vi "Find Request In VI.vi"(7 "Memory in (empty":path[](array[path]), 8 "error in":errorcluster, 10 "Level (0)":i32, 11 "VI Ref":refnum<vi>) -> (0 "error out":errorcluster, 2 "Request And Wait For Reply Names":string[](array[string]), 3 "Request Names":string[](array[string]), 5 "Memory out":path[](array[path]))   [LabVIEW 2021, in "TAF Proj Document Type.lvlib" / "Project Parser.lvlib"]
uses:
  <vilib>/Wovalab/AntiDoc/Document Type/Add-ons/LabVIEW TAF Project/Project Parser/Project Parser.lvlib
  <vilib>/Utility/traverseref.llb/TRef TravTarget.ctl
  <vilib>/Utility/traverseref.llb/VI Scripting - Traverse.lvlib
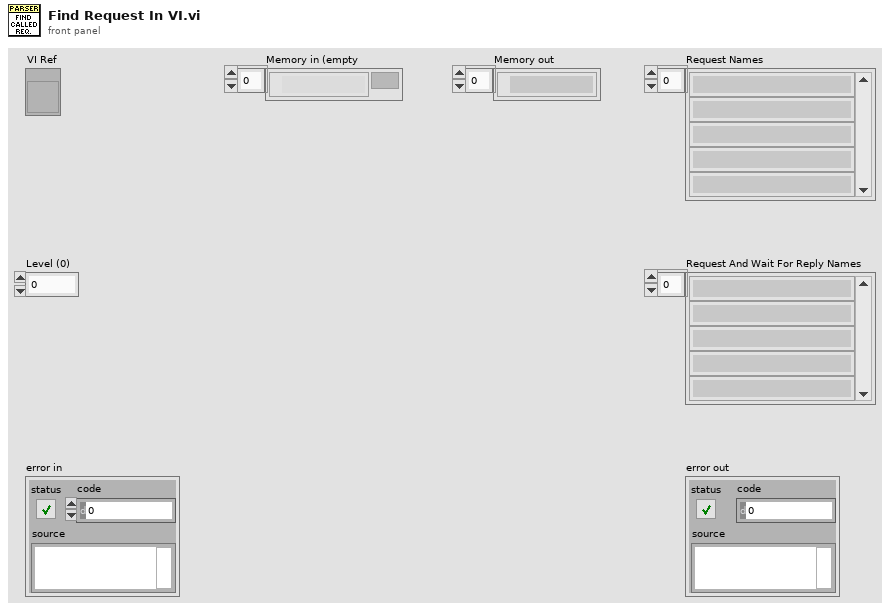
[diagram p1: front panel]
types:
  T1 = typedef "TRef TravTarget.ctl" = enum16{"FP", "BD", "Other"}
  T2 = typedef "TAF Proj Document Type.lvlib/Project Parser.lvlib/Dqmh Event Type--enum.ctl" = enum16{"Not a DQMH Event", "Request", "Request And Wait For Reply", "Broadcast"}
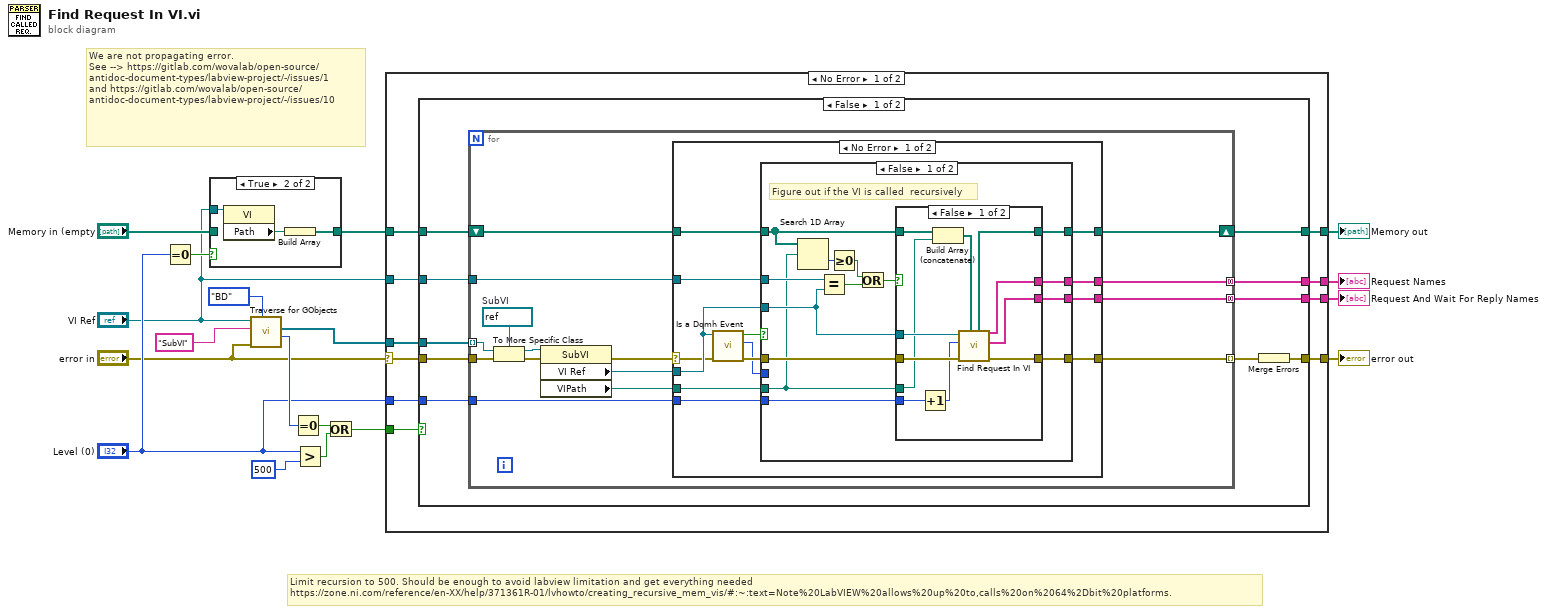
[diagram p0: block diagram]
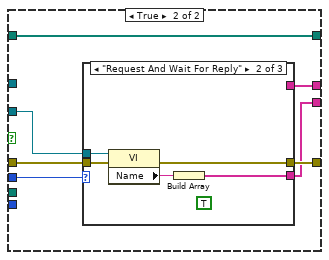
[diagram p3: hidden frame]
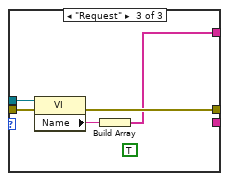
[diagram p5: hidden frame]
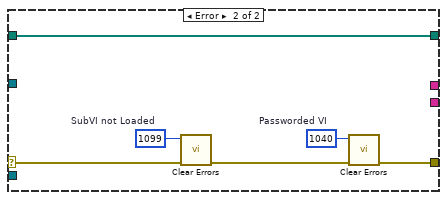
[diagram p6: hidden frame]
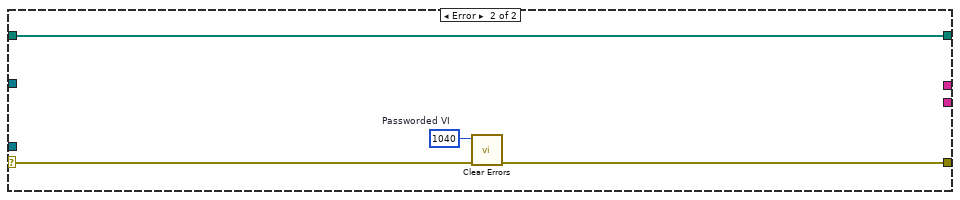
[diagram p8: hidden frame]
diagram:
  # "We are not propagating error.\nSee --> https://gitlab.com/wovalab/open-source/antidoc-document-types/labview-project/-/issues/1\nand https://gitlab.com/wovalab/open-source/antidoc-document-types/labview-project/-/issues/10"
  # "Limit recursion to 500. Should be enough to avoid labview limitation and get everything needed\nhttps://zone.ni.com/reference/en-XX/help/371361R-01/lvhowto/creating_recursive_mem_vis/#:~:text=Note%20LabVIEW%20allows%20up%20to,calls%20on%2064%2Dbit%20platforms."
  n1 = Equal To 0?(x="Level (0)") -> (x = 0?=w5:bool)
  n2 = case shown="True" w5 {
    tunnel: "Memory in (empty" -> [w19 _]
    tunnel: [w19 w20] -> w3
    tunnel: "VI Ref" -> [_ w22]
    frame False {
    }
    frame True {
      n3 = property class="VI"(reference=w22) -> ("Path"=w21:path)  [unwired: 1 in, 2 out]
      n4 = Build Array(w21) -> (w20:path[])
    }
  }
  n5 = call <vilib>:"Traverse for GObjects.vi"("Traverse Target"=TRef_TravTarget."BD", "error in (no error)"="error in", "Class Name"="SubVI", "VI Refnum"="VI Ref") -> ("# of Refs"=w12:i32, "References"=w14:refnum<vi>[])  [unwired: 4 in, 2 out]
  n6 = Equal To 0?(x=w12) -> (x = 0?=w11:bool)
  n7 = Greater?(x="Level (0)", y=500) -> (0:w10:bool)
  n8 = Or(x=w11, y=w10) -> (x .or. y?=w8:bool)
  n9 = case shown="No Error" "error in" {
    selector: "error in" -> [w31 w126]
    tunnel: [w32 w125] -> w18
    tunnel: [w30 _] -> w17
    tunnel: w14 -> [w29 _]
    tunnel: [w28 _] -> w13
    tunnel: w8 -> [w27 _]
    tunnel: [w26 w124] -> w7
    tunnel: "Level (0)" -> [w25 _]
    tunnel: w3 -> [w24 w124]
    tunnel: "VI Ref" -> [w23 _]
    frame No Error {
      n10 = case shown="False" w27 {
        tunnel: [w42 w123] -> w32
        tunnel: [w40 _] -> w30
        tunnel: w31 -> [w41 w123]
        tunnel: w29 -> [w38 _]
        tunnel: [w37 _] -> w28
        tunnel: w25 -> [w36 _]
        tunnel: w23 -> [w35 _]
        tunnel: w24 -> [w34 w122]
        tunnel: [w33 w122] -> w26
        frame False {
          n11 = for {
            tunnel: w38 -> [w54] mode=indexing
            tunnel: [w55] -> w40 mode=concatenating
            tunnel: w41 -> [w57]
            tunnel: [w43] -> w39 mode=indexing
            tunnel: [w51] -> w37 mode=concatenating
            tunnel: w36 -> [w47]
            tunnel: w35 -> [w50]
            shift-right: [w48] -> w33
            shift-left: w34 -> [w46]
            w52 = refnum<vi> refnum  # SubVI
            n12 = To More Specific Class(target class=w52, reference=w54, error in=w57) -> (specific class reference=w53:refnum<vi>, error out=w56:errorcluster)
            n13 = property class="SubVI"(reference=w53, error in=w56) -> (error out=w44:errorcluster, "VI Ref"=w45:refnum<vi>, "VIPath"=w49:path)  [unwired: 1 out]
            n14 = case shown="No Error" w44 {
              selector: w44 -> [w59 w120]
              tunnel: [w67 _] -> w55
              tunnel: [w66 _] -> w51
              tunnel: w50 -> [w65 _]
              tunnel: w49 -> [w64 _]
              tunnel: [w63 w116] -> w48
              tunnel: w47 -> [w62 _]
              tunnel: w46 -> [w61 w116]
              tunnel: w45 -> [w60 _]
              tunnel: [w58 w117] -> w43
              frame No Error {
                n15 = call <vilib>:"Is a Dqmh Event.vi"("error in"=w59, "VI Refnum"=w60) -> ("error out"=w70:errorcluster, "Event Type"=w68:T2, "Is Dqmh Event"=w69:bool)  [unwired: 7 in]
                n16 = case shown="False" w69 {
                  tunnel: w68 -> [_ w102]
                  tunnel: w60 -> [w78 w101]
                  tunnel: [w82 w100] -> w67
                  tunnel: [w83 w103] -> w58
                  tunnel: w70 -> [w84 w104]
                  tunnel: [w81 w99] -> w66
                  tunnel: w62 -> [w80 _]
                  tunnel: w65 -> [w79 _]
                  tunnel: w64 -> [w74 _]
                  tunnel: [w76 w98] -> w63
                  tunnel: w61 -> [w71 w98]
                  frame False {
                    # "Figure out if the VI is called  recursively"
                    n17 = Search 1D Array(1D array=w71, element=w74) -> (index of element=w73:i32)  [unwired: 1 in]
                    n18 = Equal?(x=w79, y=w78) -> (x = y?=w77:bool)
                    n19 = Greater Or Equal To 0?(x=w73) -> (x >= 0?=w72:bool)
                    n20 = Or(x=w72, y=w77) -> (x .or. y?=w75:bool)
                    n21 = case shown="False" w75 {
                      tunnel: w84 -> [w95 w97]
                      tunnel: [w94 w97] -> w83
                      tunnel: [w93 _] -> w82
                      tunnel: [w92 _] -> w81
                      tunnel: w80 -> [w91 _]
                      tunnel: w78 -> [w89 _]
                      tunnel: w74 -> [w88 _]
                      tunnel: [w85 w96] -> w76
                      tunnel: w71 -> [w87 w96]
                      frame False {
                        n22 = Increment(x=w91) -> (x+1=w90:i32)
                        n23 = Build Array (concatenate)(w87, w88) -> (w86:path[])
                        n24 = call <vilib>:"Find Request In VI.vi"("Memory in (empty"=w86, "error in"=w95, "Level (0)"=w90, "VI Ref"=w89) -> ("error out"=w94:errorcluster, "Request And Wait For Reply Names"=w93:string[], "Request Names"=w92:string[], "Memory out"=w85:path[])  [unwired: 4 in]
                      }
                      frame True {
                        # "Stop recursion call"
                      }
                    }
                  }
                  frame True {
                    n25 = case shown="\"Request And Wait For Reply\"" w102 {
                      tunnel: w101 -> [_ w108 w113]
                      tunnel: [_ w106 _] -> w100
                      tunnel: w104 -> [w105 w110 w115]
                      tunnel: [w105 w109 w114] -> w103
                      tunnel: [_ _ w111] -> w99
                      frame "Not a DQMH Event", "Broadcast" {
                      }
                      frame "Request And Wait For Reply" {
                        (unwired) TRUE
                        n26 = property class="VI"(reference=w108, error in=w110) -> (error out=w109:errorcluster, "Name"=w107:string)  [unwired: 1 out]
                        n27 = Build Array(w107) -> (w106:string[])
                      }
                      frame "Request" {
                        (unwired) TRUE
                        n28 = property class="VI"(reference=w113, error in=w115) -> (error out=w114:errorcluster, "Name"=w112:string)  [unwired: 1 out]
                        n29 = Build Array(w112) -> (w111:string[])
                      }
                    }
                  }
                }
              }
              frame Error {
                w119 = 1040  # Passworded VI
                w121 = 1099  # SubVI not Loaded
                n30 = call <vilib>:"Clear Errors.vi"("error in (no error)"=w120, "specific error code to clear (0: all)"=w121) -> ("error out"=w118:errorcluster)  [unwired: 4 in, 1 out]
                n31 = call <vilib>:"Clear Errors.vi"("error in (no error)"=w118, "specific error code to clear (0: all)"=w119) -> ("error out"=w117:errorcluster)  [unwired: 4 in, 1 out]
              }
            }
          }
          n32 = Merge Errors(w39) -> (w42:errorcluster)
        }
        frame True {
          # "Stop recursion call"
        }
      }
    }
    frame Error {
      w127 = 1040  # Passworded VI
      n33 = call <vilib>:"Clear Errors.vi"("error in (no error)"=w126, "specific error code to clear (0: all)"=w127) -> ("error out"=w125:errorcluster)  [unwired: 4 in, 1 out]
    }
  }
  "Request And Wait For Reply Names" <- w17
  "error out" <- w18
  "Request Names" <- w13
  "Memory out" <- w7
